vi "CRC校验.vi"(1 "要校验的字符串（十六进制显示）":string) -> (0 "CRC32效验码输出":string)   [LabVIEW 2016, in "数据传输系统.lvlib" / "自动更新.lvlib" / "TCP文件传输系统.lvlib" / "TCP接收文件.lvlib"]
panel:
  out "输出字符串":string
  in  "停止":bool
  out "CRC校验":bool
  out "PSI/SI表":u8[](array[numeric]) format="%.0x"
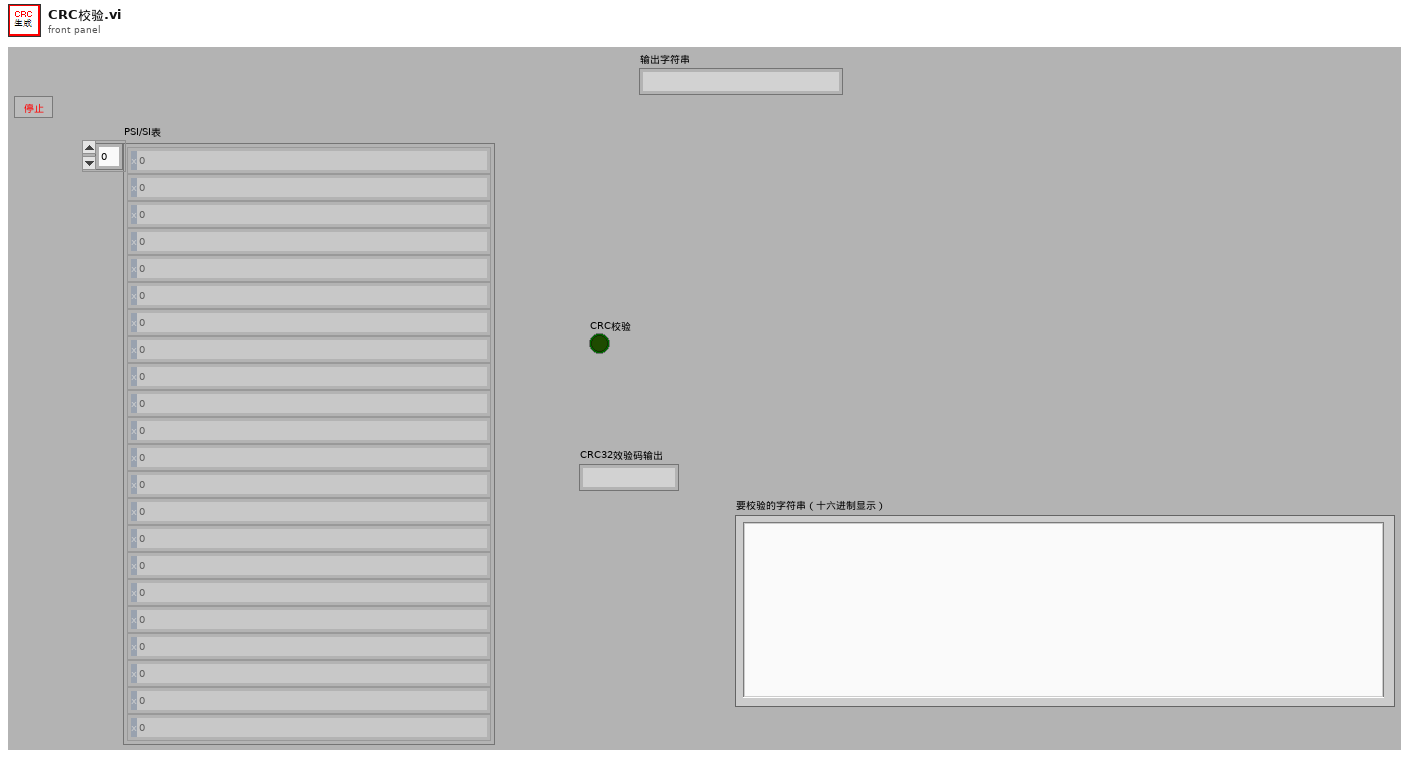
[diagram p1: front panel]
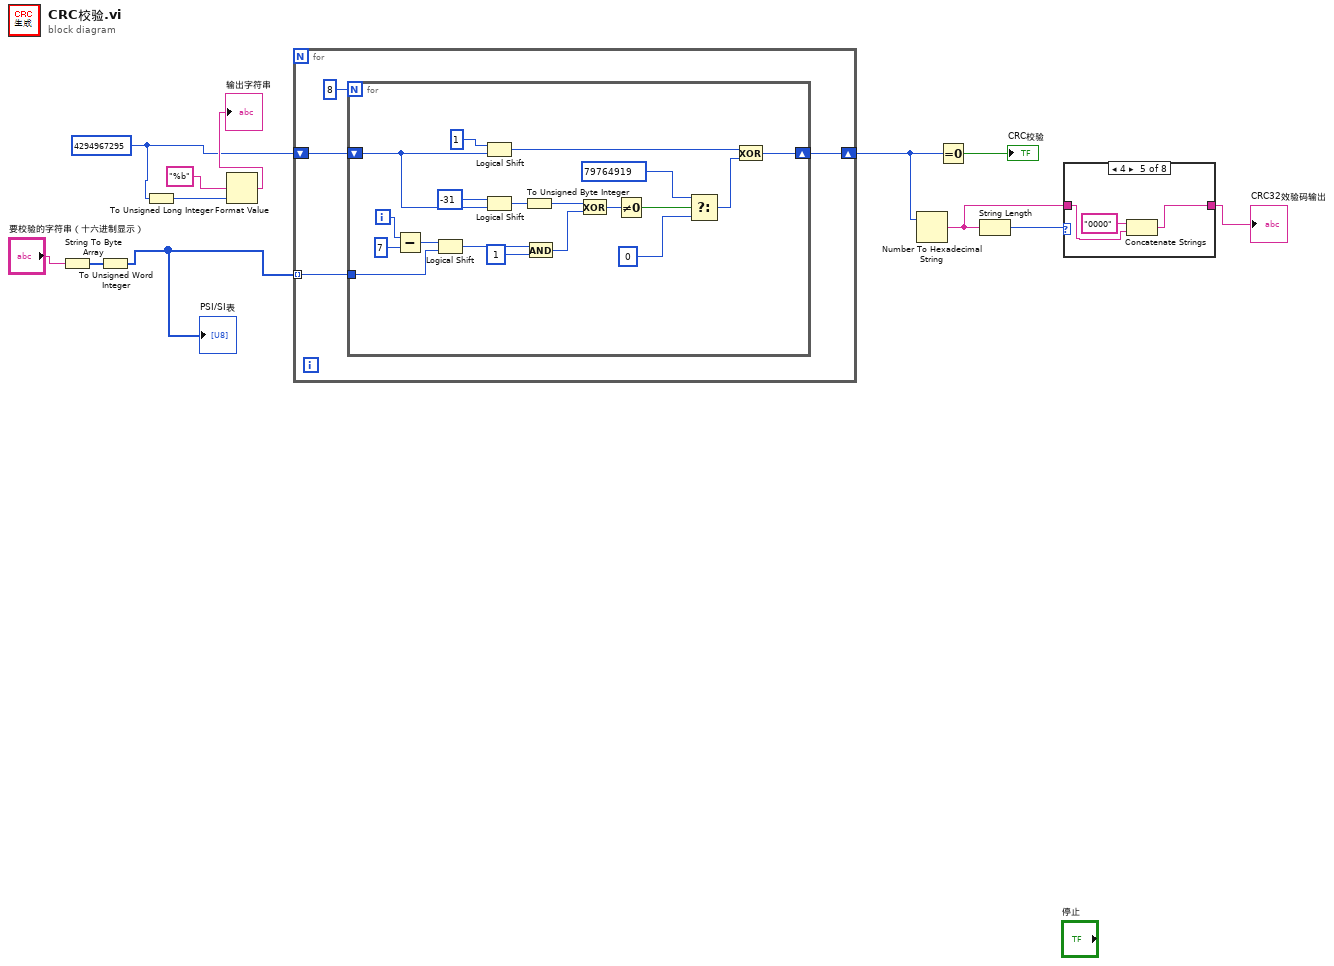
[diagram p0: block diagram]
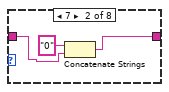
[diagram p3: hidden frame]
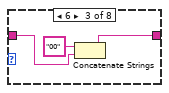
[diagram p4: hidden frame]
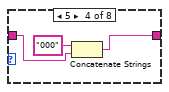
[diagram p5: hidden frame]
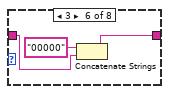
[diagram p6: hidden frame]
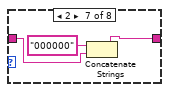
[diagram p7: hidden frame]
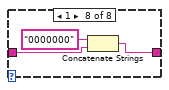
[diagram p8: hidden frame]
diagram:
  w6 = u32 4294967295
  n1 = String To Byte Array(string="要校验的字符串（十六进制显示）") -> (unsigned byte array=w11:u8[])
  n2 = To Unsigned Word Integer(number=w11) -> (unsigned 16bit integer=w9:u16[])
  "PSI/SI表" <- w9
  n3 = To Unsigned Long Integer(number=w6) -> (unsigned 32bit integer=w5:u32)
  n4 = Format Value(format string="%b" ("字符串(\"\")"), value (0)=w5) -> (output string=→"输出字符串":string)  [unwired: 1 in]
  n5 = for {
    tunnel: w9 -> [w16] mode=indexing
    shift-right: [w14] -> w10
    shift-left: w6 -> [w15]
    n6 = for {
      N: 8 -> [_]
      tunnel: w16 -> [w32]
      shift-right: [w34] -> w14
      shift-left: w15 -> [w26]
      i -> [w18]
      n7 = Subtract(x=w18, y=7) -> (x-y=w33:i32)
      n8 = Logical Shift(y=w33, x=w32) -> (x << y=w31:u16)
      n9 = Logical Shift(y=1 ("x"), x=w26) -> (x << y=w35:u32)
      n10 = Logical Shift(y=-31 ("x"), x=w26) -> (x << y=w25:u32)
      n11 = To Unsigned Byte Integer(number=w25) -> (unsigned 8bit integer=w24:u8)
      n12 = And(x=w31, y=u8 1) -> (x .and. y?=w29:u16)
      n13 = Exclusive Or(1:w29, 2:w24) -> (0:w23:u16)
      n14 = Not Equal To 0?(x=w23) -> (x != 0?=w22:bool)
      n15 = Select(t=u32 79764919, s=w22, f=u32 0) -> (s? t:f=w19:u32)
      n16 = Exclusive Or(1:w19, 2:w35) -> (0:w34:u32)
    }
  }
  n17 = Number To Hexadecimal String(2:w10) -> (0:w2:string)  [unwired: 1 in]
  n18 = Equal To 0?(x=w10) -> (x = 0?=→"CRC校验":bool)
  n19 = String Length(string=w2) -> (length=w4:i32)
  n20 = case shown="4" w4 {
    tunnel: [w36 w39 w40 w44 w46 w49 w52 w55] -> w3
    tunnel: w2 -> [w36 w37 w41 w43 w47 w50 w53 w56]
    frame 8, Default {
    }
    frame 7 {
      n21 = Concatenate Strings("0" ("字符串"), w37) -> (w39:string)
    }
    frame 6 {
      n22 = Concatenate Strings("00" ("字符串"), w41) -> (w40:string)
    }
    frame 5 {
      n23 = Concatenate Strings("000" ("字符串"), w43) -> (w44:string)
    }
    frame 4 {
      n24 = Concatenate Strings("0000" ("字符串"), w47) -> (w46:string)
    }
    frame 3 {
      n25 = Concatenate Strings("00000" ("字符串"), w50) -> (w49:string)
    }
    frame 2 {
      n26 = Concatenate Strings("000000" ("字符串"), w53) -> (w52:string)
    }
    frame 1 {
      n27 = Concatenate Strings("0000000" ("字符串"), w56) -> (w55:string)
    }
  }
  "CRC32效验码输出" <- w3
